vi "Get Relative Humidity.vi"(8 "error in (no error)":errorcluster, 11 "Sensor General Class in":refnum<class "Sensor General Class.lvclass">) -> (0 "error out":errorcluster, 2 "relative humidity":sgl, 3 "Sensor General Class out":refnum<class "Sensor General Class.lvclass">)   [LabVIEW 2020, in "Sensor General Class.lvclass"]
uses:
  Sensor General Class.lvclass
  Data Enum.ctl
  Sensor General Class.lvclass/Sensor General Class.ctl
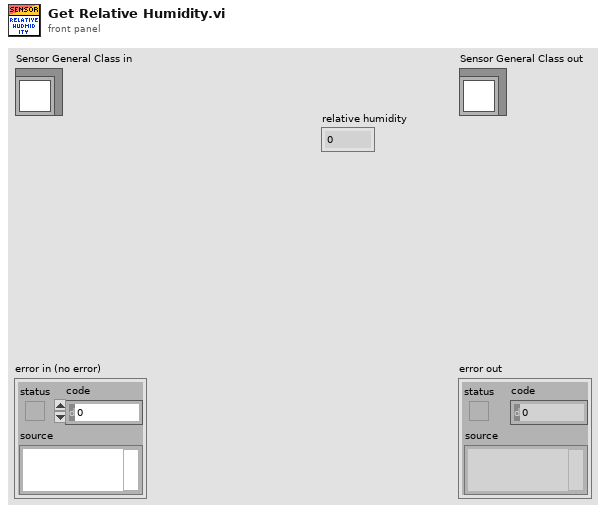
[diagram p1: front panel]
types:
  T1 = typedef "Sensor General Class.lvclass/Data Enum.ctl" = enum16{"p_bar", "p_MPa", "p_Pa", "p_kPa", "p_psi", "p_H/cm^2", "t_C", "t_K", "t_F", "rho_g/l", "rho_kg/m^3", "p20_bar", "related p20_bar", "p20_MPa", "related p20_MPa", "Tf_SF6", "Td_sf6", "tank Tf_SF6", "tank Td_SF6", "Tf_N2", "Td_N2", "tank Tf_N2", "tank Td_N2", "ppm_v SF6", "ppm_w SF6", "ppm_v N2", "ppm_w N2", "rH", "errors"}
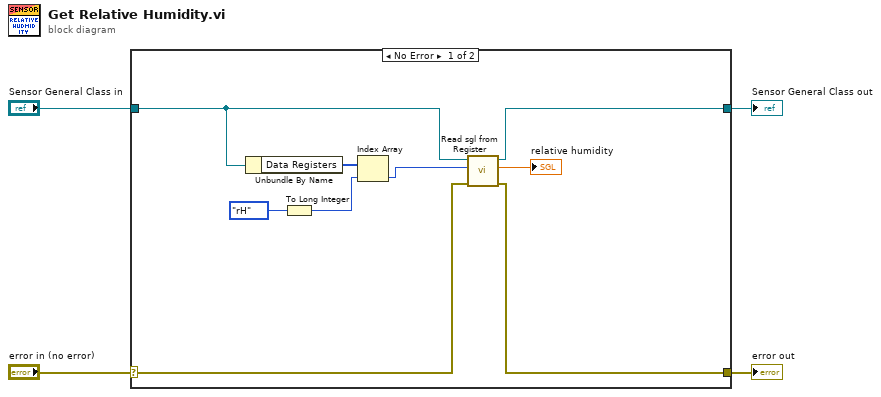
[diagram p0: block diagram]
diagram:
  n1 = case shown="No Error" "error in (no error)" {
    selector: "error in (no error)" -> [w13 w15]
    tunnel: [w12 w15] -> w3
    tunnel: [w5 w14] -> w1
    tunnel: "Sensor General Class in" -> [w11 w14]
    frame No Error {
      n2 = Unbundle By Name(w11) -> ("Data Registers"=w10:u16[])
      n3 = To Long Integer(number=Data_Enum."rH" ("Data Enum")) -> (32bit integer=w8:i32)
      n4 = Index Array(array=w10, index=w8) -> (element=w7:u16)
      n5 = call-dynamic "Read sgl from Register.vi"("error in (no error)"=w13, "Start Register"=w7, "Sensor General Class in"=w11) -> ("error out"=w12:errorcluster, "Data"=→"relative humidity":sgl, "Sensor General Class out"=w5:refnum<class "Sensor General Class.lvclass">)  [unwired: 6 in]
    }
    frame Error {
    }
  }
  "error out" <- w3
  "Sensor General Class out" <- w1
